vi "FileNamer_SM.vi"() -> ()   [LabVIEW 2024]
uses:
  TypeDefs/comic--cluster.ctl
  <userlib>/_OpenG.lib/array/array.llb/Remove Duplicates from 1D Array (String)__ogtk.vi
  <userlib>/_OpenG.lib/array/array.llb/Sort 1D Array (String)__ogtk.vi
  <userlib>/_OpenG.lib/file/file.llb/Strip Path Extension - String__ogtk.vi
  <userlib>/_OpenG.lib/array/array.llb/Remove Duplicates from 1D Array (DBL)__ogtk.vi
  <userlib>/_OpenG.lib/file/file.llb/Strip Path Extension - Path__ogtk.vi
  <userlib>/_OpenG.lib/array/array.llb/openg_array.lvlib
  <vilib>/httpClient/LabVIEWHTTPClient.lvlib
  <vilib>/addons/_JKI.lib/Serialization/JSON/JKI JSON Serialization.lvlib
  <userlib>/_OpenG.lib/file/file.llb/openg_file.lvlib
  <userlib>/_OpenG.lib/string/string.llb/openg_string.lvlib
panel:
  out "Available?":bool
  out "missing json":string
  out "missing current":string
  in  "Create New Folder":bool
  in  "json file path":path
  in  "Rename Available":bool
  out "json count":string
  out "current count":string
  in  "Rename Selected":bool
  in  "Delete from json":bool
  out "web cover":picture
  out "Local Cover":picture
  out "totals match":bool
  in  "Rename All":bool
  out "synced":bool
  in  "Rename Selected":bool
  in  "Folders":i32(listbox)
  in  "Parent Path":path
  in  "From json":i32(listbox)
  in  "Current":i32(listbox)
  in  "OK":bool
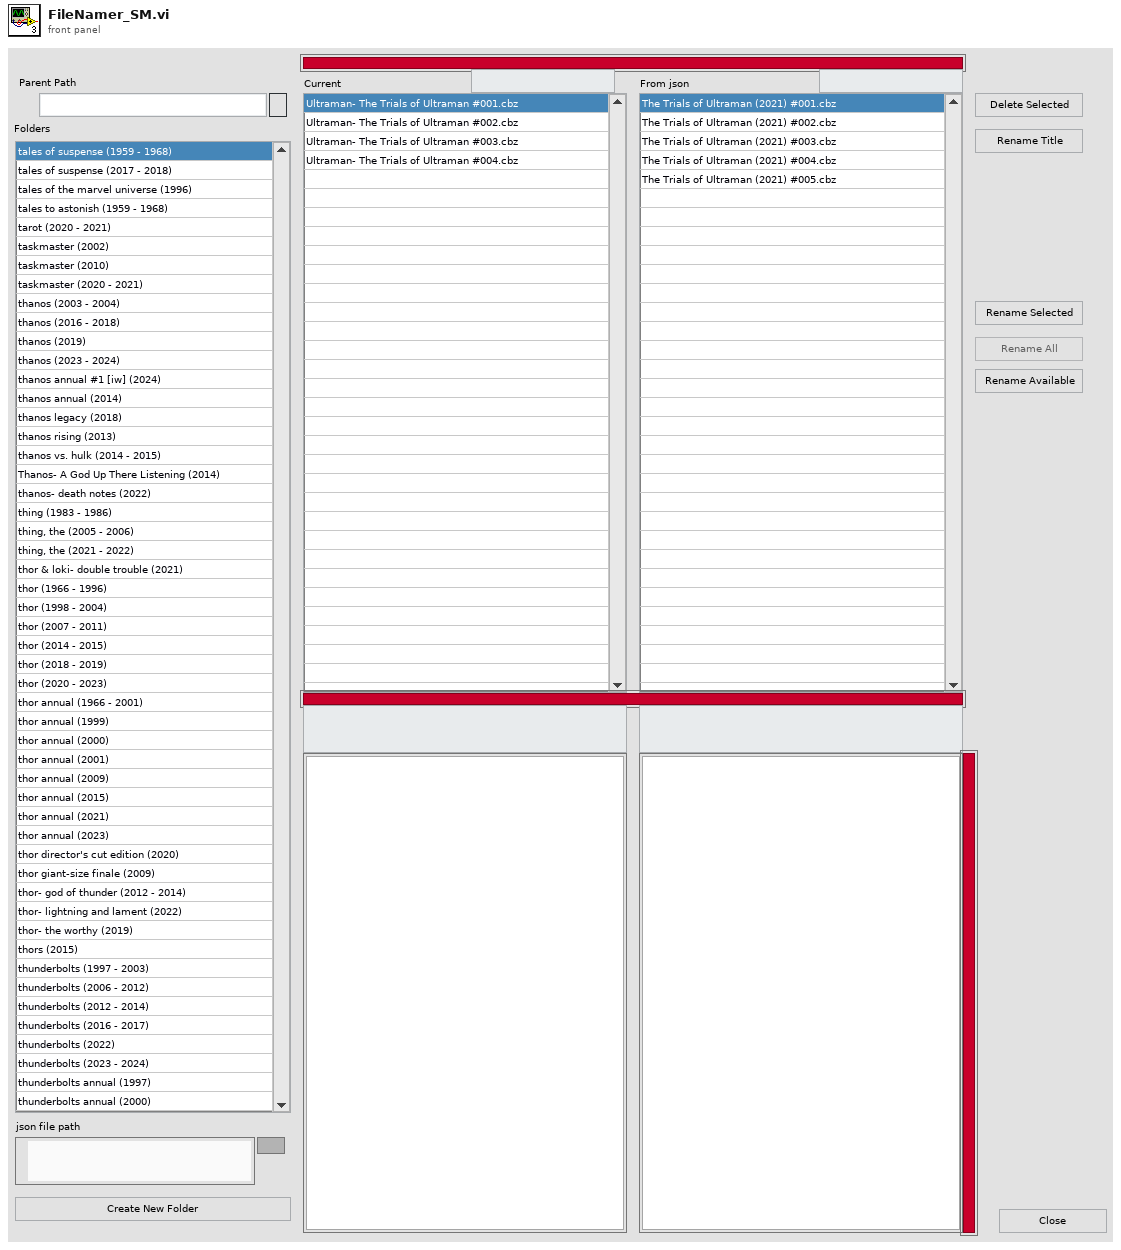
[diagram p1: front panel]
types:
  T1 = enum32{"Invalid", "Standard", "Closed", "Hidden", "Minimized", "Maximized"}
  T2 = enum32{"invalid app kind", "Development System", "Run Time System", "Student Edition", "Embedded LabVIEW", "Evaluation", "Custom"}
  T3 = enum16{"open", "replace", "create", "open or create", "replace or create", "replace or create with confirmation"}
  T4 = enum8{"Enabled", "Disabled", "Disabled and Grayed Out"}
  T5 = typedef "comic--cluster.ctl" = cluster{"id":i32, "digitalId":i32, "title":string, "issueNumber":i32, "variantDescription":string, "description":string, "modified":variant, "upc":string, "format":string, "pageCount":i32, "resourceURI":string, "urls":cluster{"type":string, "url":string}[], "series":cluster{"resourceURI":string, "name":string}, "dates":cluster{"type":string, "date":string}[], "prices":cluster{"price":dbl, "type":string}[], "thumbnail":cluster{"path":string, "extension":string}, "images":cluster{"path":string, "extension":string}[], "creators":cluster{"available":i32, "returned":i32, "collectionURI":string, "items":cluster{"resourceURI":string, "name":string, "role":string}[]}, "characters":cluster{"available":i32, "returned":i32, "collectionURI":string, "items":cluster{"resourceURI":string, "name":string}[]}, "stories":cluster{"available":i32, "returned":i32, "collectionURI":string, "items":cluster{"resourceURI":string, "name":string, "type":string}[]}, "events":cluster{"available":i32, "returned":i32, "collectionURI":string, "items":cluster{"resourceURI":string, "name":string}[]}}
  T6 = cluster{"Core":cluster{"Current VI Reference":refnum<vi>, "Close Panel on Exit?":bool}, "current folder":path, "comic jsons":T5[], "local working folder":path, "web working folder":path, "json present":bool, "display web":bool}
  T7 = cluster{"Current VI Reference":refnum<vi>, "Close Panel on Exit?":bool}
  T8 = typedef "comics.reply--cluster.ctl" = cluster{"code":i32, "status":string, "etag":string, "data":cluster{"offset":i32, "limit":i32, "total":i32, "count":i32, "results":T5[]}}
  T9 = typedef "imagedata.ctl" = cluster{"image type":i32, "image depth":i32, "image":u8[], "mask":u8[], "colors":u32[], "Rectangle":cluster{"left":i16, "top":i16, "right":i16, "bottom":i16}}
  T10 = typedef "LVBoundsTypeDef.ctl" = cluster{"Width":u32, "Height":u32}
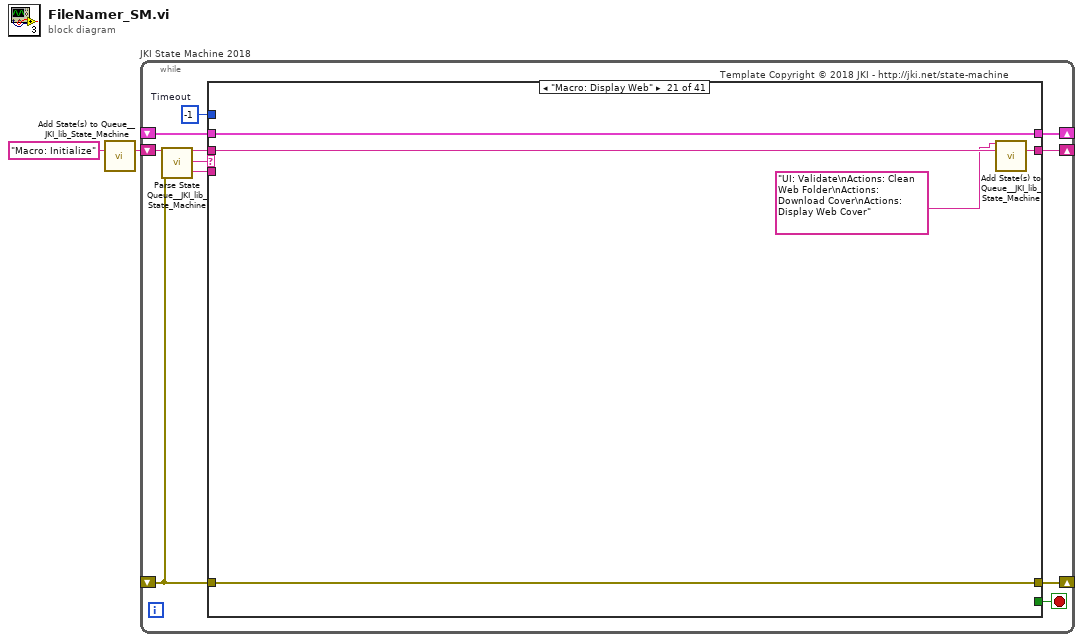
[diagram p0: block diagram]
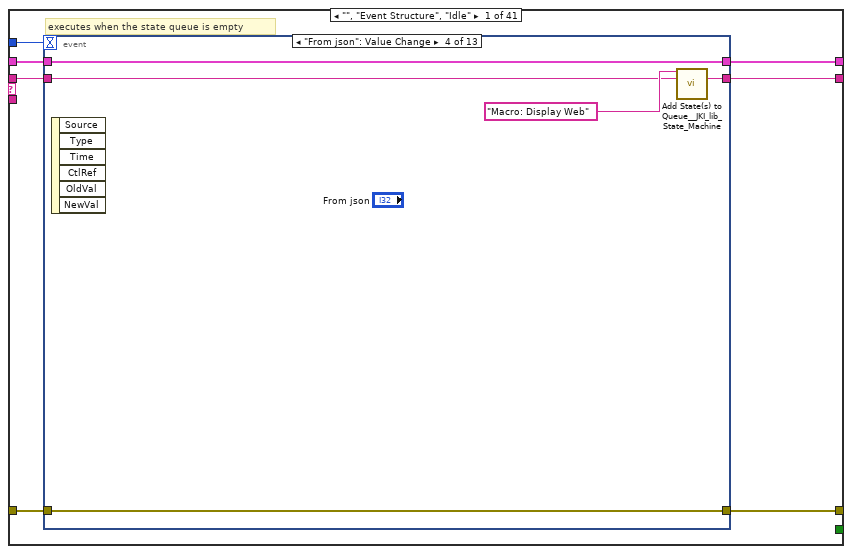
[diagram p2: hidden frame]
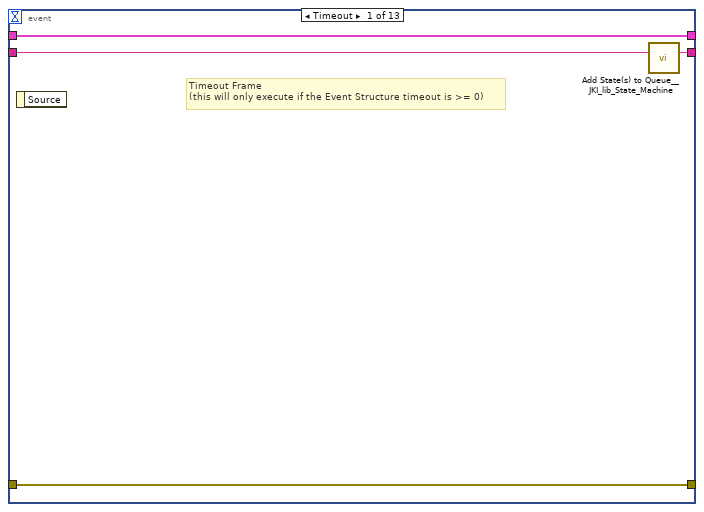
[diagram p3: hidden frame]
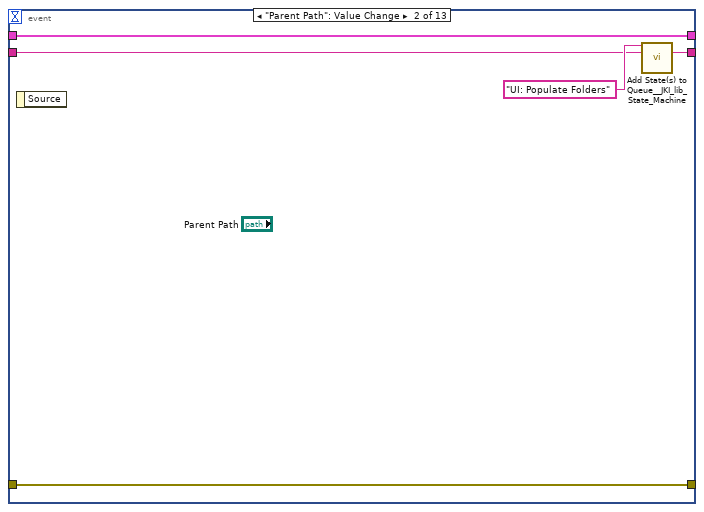
[diagram p4: hidden frame]
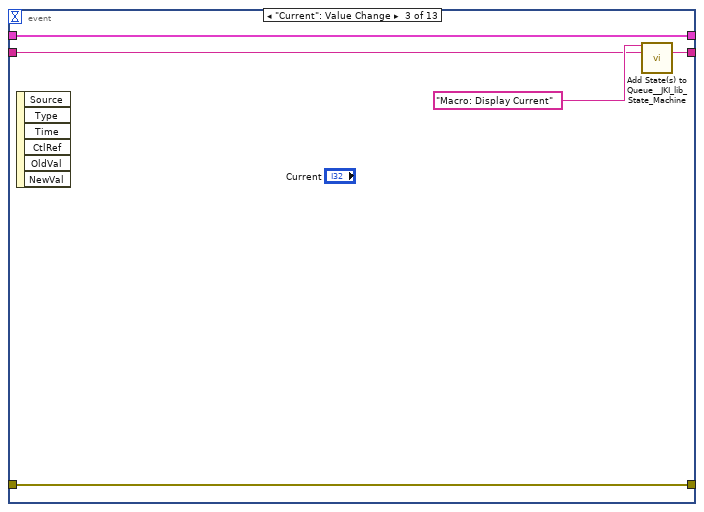
[diagram p5: hidden frame]
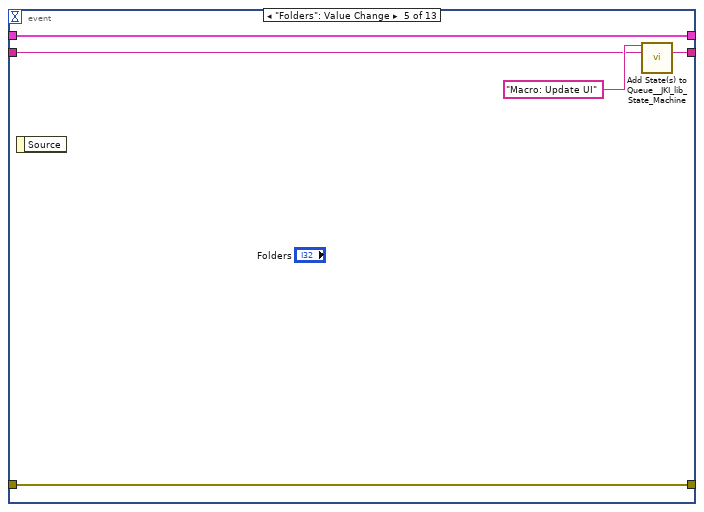
[diagram p6: hidden frame]
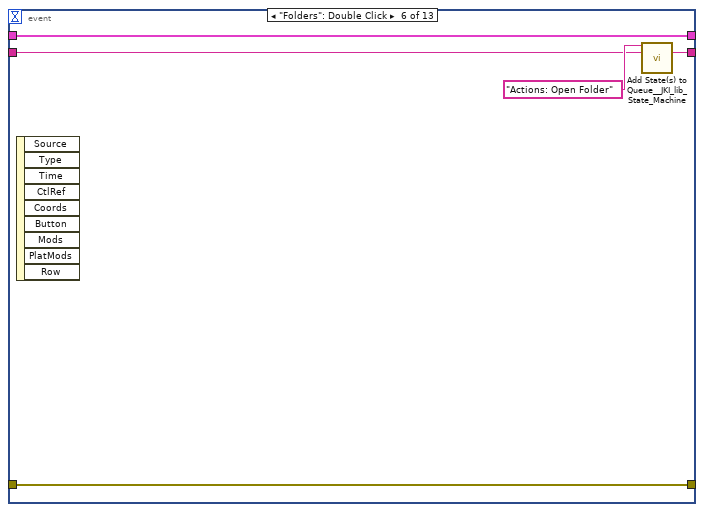
[diagram p7: hidden frame]
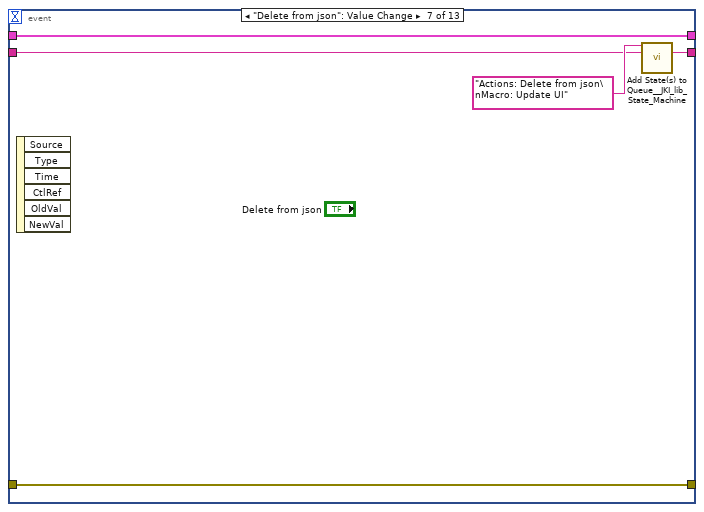
[diagram p8: hidden frame]
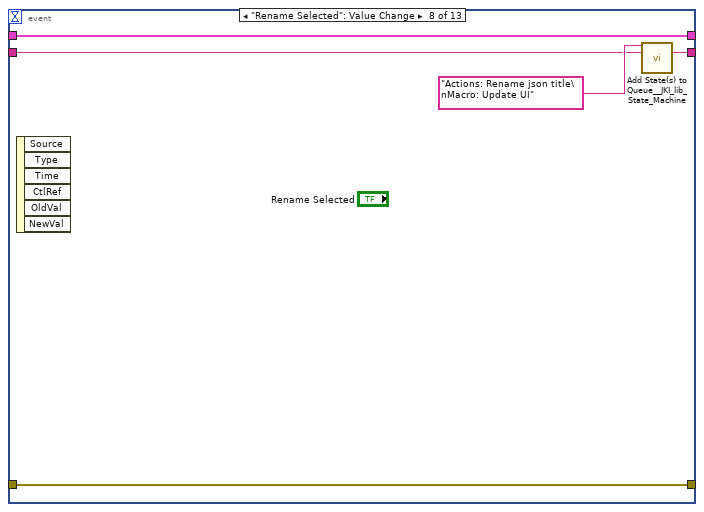
[diagram p9: hidden frame]
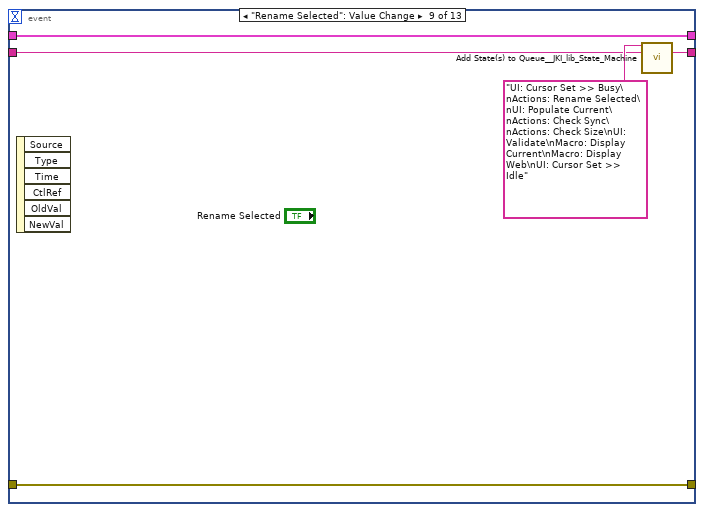
[diagram p10: hidden frame]
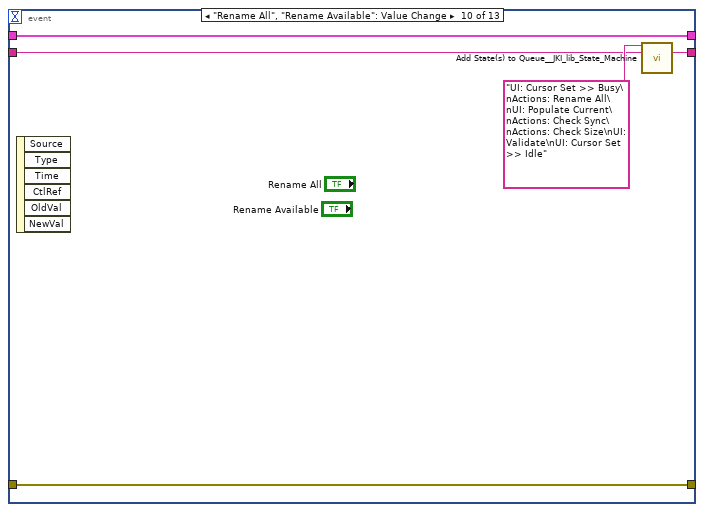
[diagram p11: hidden frame]
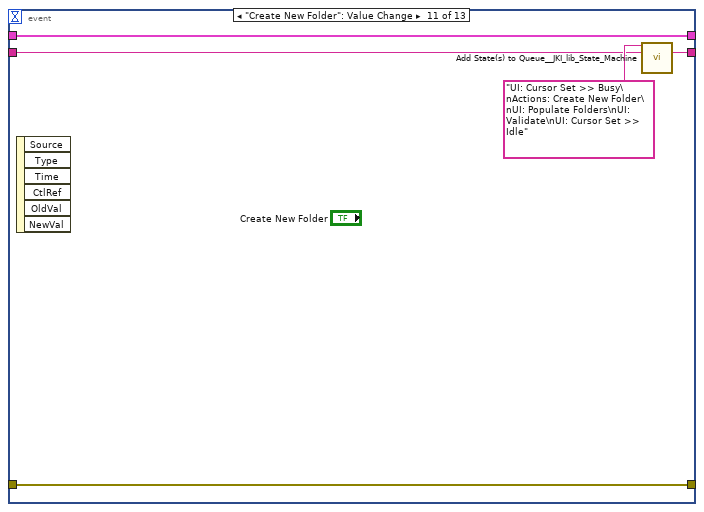
[diagram p12: hidden frame]
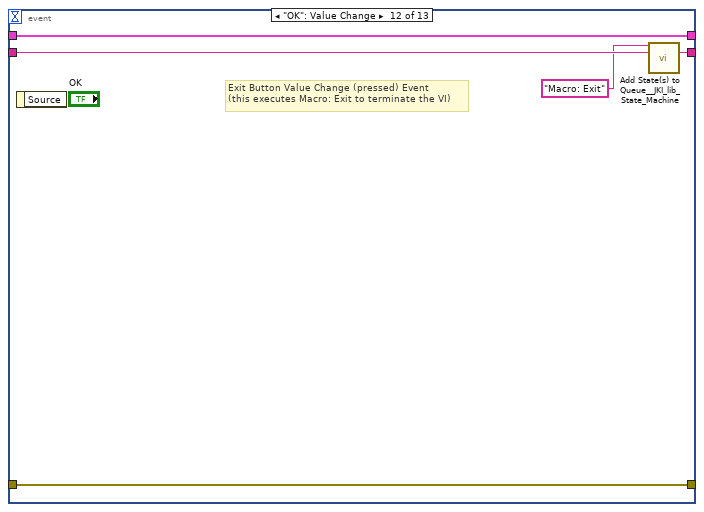
[diagram p13: hidden frame]
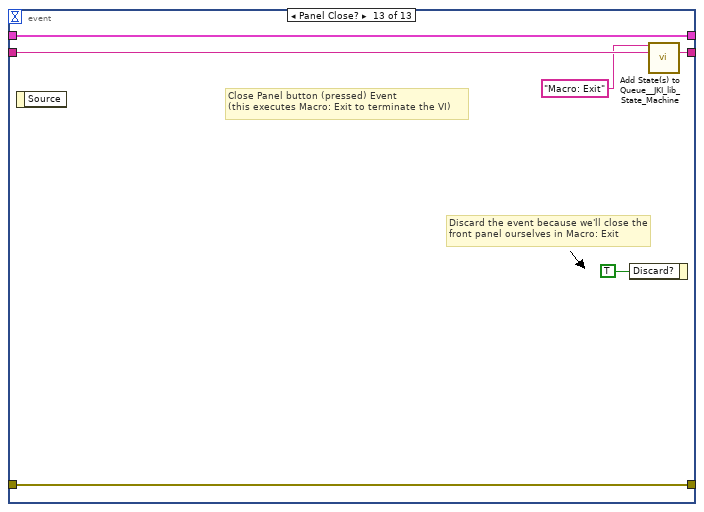
[diagram p14: hidden frame]
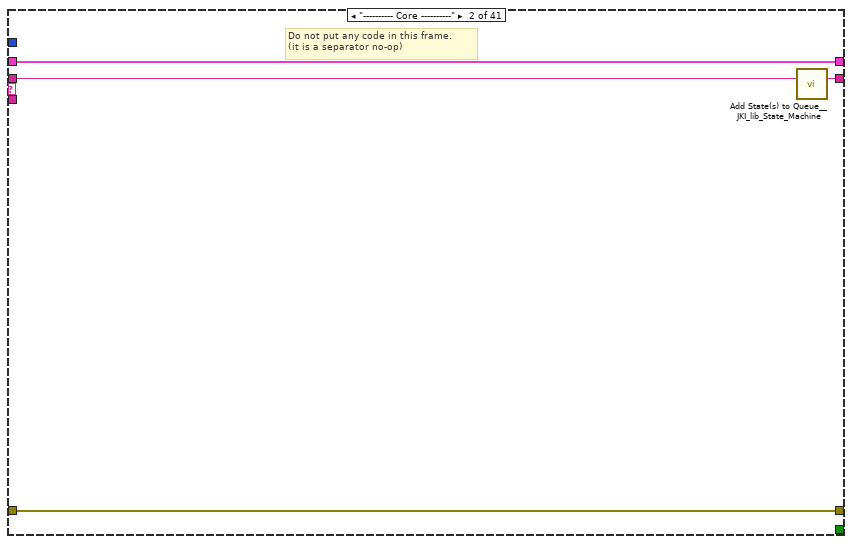
[diagram p15: hidden frame]
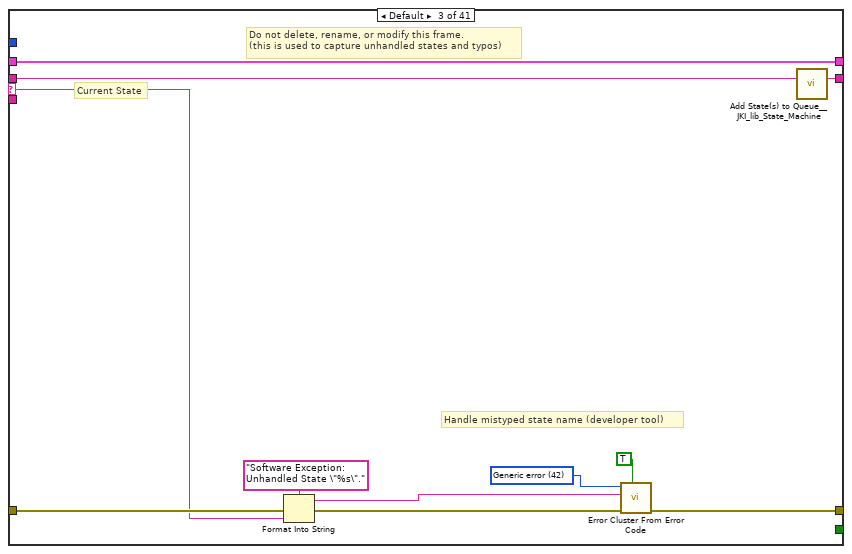
[diagram p16: hidden frame]
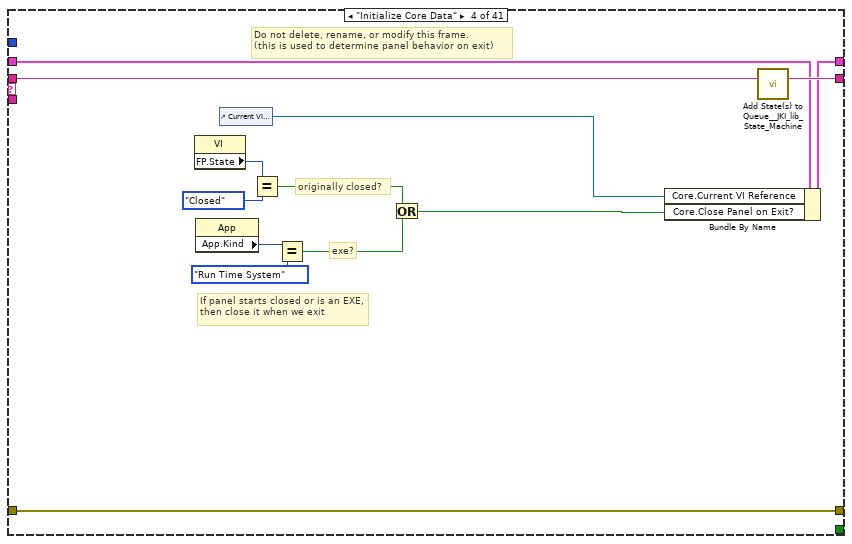
[diagram p17: hidden frame]
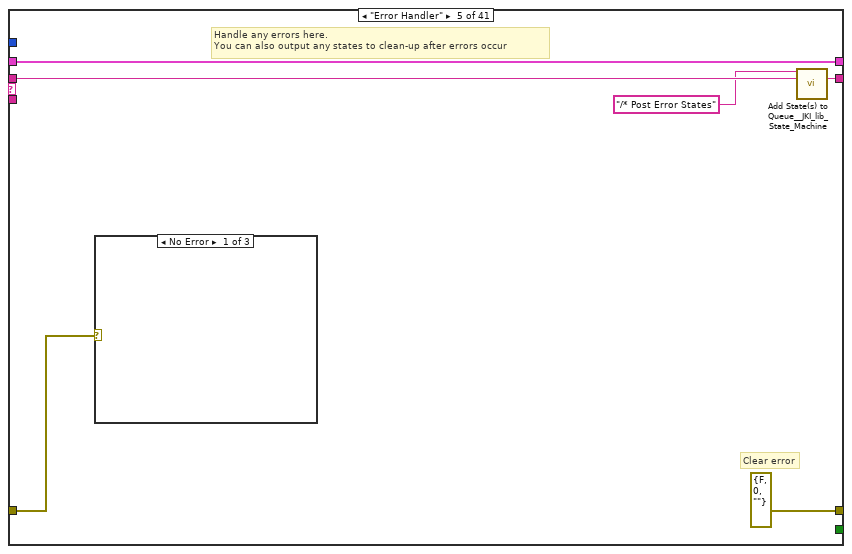
[diagram p18: hidden frame]
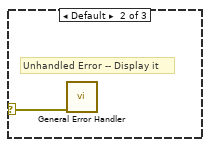
[diagram p19: hidden frame]
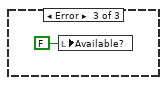
[diagram p20: hidden frame]
diagram:
  n1 = call <vilib>:"Add State(s) to Queue__JKI_lib_State_Machine.vi"("State(s) in (\"\")"="Macro: Initialize") -> ("States Out"=w2:string)  [unwired: 14 in]
  n2 = while "JKI State Machine 2018" {
    shift-right: [w6] -> _
    shift-left: _ -> [w5]
    shift-right: [w9] -> _
    shift-left: _ -> [w3]
    shift-right: [w8] -> _
    shift-left: w2 -> [w10]
    stop <- w7 stop-if-true
    w4 = -1  # Timeout
    # "Template Copyright © 2018 JKI - http://jki.net/state-machine"
    n3 = call <vilib>:"Parse State Queue__JKI_lib_State_Machine.vi"("State Queue"=w10, "Error In (no error)"=w3) -> ("Remaining States"=w12:string, "Current State"=w13:string, "Arguments"=w11:string)  [unwired: 11 in]
    n4 = case shown="\"Macro: Display Web\"" w13 {
      selector: w13 -> [_ _ w90 _ _ _ _ _ _ _ _ _ _ _ _ _ _ _ _ _ _ _ _ _ _ _ _ _ _ _ _ _ _ _ _ _ _ _ _ _ _]
      tunnel: w12 -> [w20 w89 w94 w113 w119 w126 w130 w141 w147 w151 w162 w171 w201 w237 w246 w267 w285 w296 w365 w370 w375 w380 w385 w395 w399 w405 w426 w487 w518 w527 w567 w612 w645 w672 w678 w684 w702 w721 w744 w758 w780]
      tunnel: w11 -> [_ _ _ _ _ _ _ _ _ _ _ _ _ _ _ _ w280 w290 _ _ _ _ _ _ _ _ _ _ _ _ _ _ _ _ _ _ _ _ _ _ _]
      tunnel: w5 -> [w18 w86 w92 w106 w116 w124 w127 _ w142 w148 w156 w165 w196 w231 w244 w262 w283 w292 w362 w367 w372 w377 w382 w392 w396 w403 w423 w485 w513 w525 w558 w610 w643 w662 w674 w680 w693 w715 w738 w755 w777]
      tunnel: [w17 w87 w96 w110 errorcluster {"status"=FALSE, "code"=0, "source"=""} ("error out") w123 w128 w138 w143 w149 w157 w166 w199 w224 w239 w247 w281 w293 w363 w368 w373 w378 w383 w393 w397 w400 w424 w484 w496 w523 w559 w592 w631 w663 w676 w682 w694 w716 w739 w753 w775] -> w9
      tunnel: w3 -> [w16 w87 w95 w110 w114 w123 w128 w138 w144 w149 w160 w168 w198 w226 w242 w250 w282 w294 w363 w368 w373 w378 w383 w393 w397 w401 w424 w478 w509 w522 w562 w608 w629 w658 w675 w681 w695 w719 w737 w756 w778]
      tunnel: [w19 w88 w93 w112 w118 w125 w129 w140 w146 w150 w161 w170 w200 w236 w245 w266 w284 w295 w364 w369 w374 w379 w384 w394 w398 w404 w425 w486 w517 w526 w566 w611 w644 w671 w677 w683 w701 w720 w743 w757 w779] -> w8
      tunnel: [_ _ _ _ _ TRUE _ _ _ _ _ _ _ _ _ _ _ _ _ _ _ _ _ _ _ _ _ _ _ _ _ _ _ _ _ _ _ _ _ _ _] -> w7
      tunnel: [w15 w86 w92 w111 w116 w124 w127 w139 w142 w148 w156 w165 w195 w230 w244 w261 w283 w292 w362 w367 w372 w377 w382 w392 w396 w403 w423 w485 w512 w524 w557 w610 w643 w662 w674 w680 w692 w715 w738 w755 w777] -> w6
      tunnel: w4 -> [w14 _ _ _ _ _ _ _ _ _ _ _ _ _ _ _ _ _ _ _ _ _ _ _ _ _ _ _ _ _ _ _ _ _ _ _ _ _ _ _ _]
      frame "", "Event Structure", "Idle" {
        # "executes when the state queue is empty"
        n5 = event shown="[3] \"From json\": Value Change" {
          selector: _ -> [_ _ _ _ _ _ _ _ _ _ _ _ _]
          dyn-events: _ -> [_ _ _ _ _ _ _ _ _ _ _ _ _]
          timeout: w14 -> [_ _ _ _ _ _ _ _ _ _ _ _ _]
          tunnel: w20 -> [w24 w27 w32 w37 w42 w47 w52 w57 w62 w67 w72 w79 w85]
          tunnel: [w23 w26 w31 w36 w41 w46 w51 w56 w61 w66 w71 w78 w84] -> w19
          tunnel: w18 -> [w21 w28 w33 w38 w43 w48 w53 w58 w63 w68 w73 w76 w82]
          tunnel: [w22 w25 w30 w35 w40 w45 w50 w55 w60 w65 w70 w77 w83] -> w17
          tunnel: w16 -> [w22 w25 w30 w35 w40 w45 w50 w55 w60 w65 w70 w77 w83]
          tunnel: [w21 w28 w33 w38 w43 w48 w53 w58 w63 w68 w73 w76 w82] -> w15
          event Timeout {
            # "Timeout Frame\n(this will only execute if the Event Structure timeout is >= 0)"
            n6 = event-data() -> ()  [unwired: 1 in, 1 out]
            n7 = call <vilib>:"Add State(s) to Queue__JKI_lib_State_Machine.vi"("State(s) in (\"\")"=w24) -> ("States Out"=w23:string)  [unwired: 14 in]
          }
          event "Parent Path": Value Change {
            n8 = event-data() -> ()  [unwired: 1 in, 1 out]
            n9 = call <vilib>:"Add State(s) to Queue__JKI_lib_State_Machine.vi"("State(s) in Front (\"\")"="UI: Populate Folders", "State(s) in (\"\")"=w27) -> ("States Out"=w26:string)  [unwired: 13 in]
          }
          event "Current": Value Change {
            n10 = event-data() -> ()  [unwired: 1 in, 6 out]
            n11 = call <vilib>:"Add State(s) to Queue__JKI_lib_State_Machine.vi"("State(s) in Front (\"\")"="Macro: Display Current", "State(s) in (\"\")"=w32) -> ("States Out"=w31:string)  [unwired: 13 in]
          }
          event "From json": Value Change {
            n12 = event-data() -> ()  [unwired: 1 in, 6 out]
            n13 = call <vilib>:"Add State(s) to Queue__JKI_lib_State_Machine.vi"("State(s) in Front (\"\")"="Macro: Display Web", "State(s) in (\"\")"=w37) -> ("States Out"=w36:string)  [unwired: 13 in]
          }
          event "Folders": Value Change {
            n14 = event-data() -> ()  [unwired: 1 in, 1 out]
            n15 = call <vilib>:"Add State(s) to Queue__JKI_lib_State_Machine.vi"("State(s) in Front (\"\")"="Macro: Update UI", "State(s) in (\"\")"=w42) -> ("States Out"=w41:string)  [unwired: 13 in]
          }
          event "Folders": Double Click {
            n16 = event-data() -> ()  [unwired: 1 in, 9 out]
            n17 = call <vilib>:"Add State(s) to Queue__JKI_lib_State_Machine.vi"("State(s) in Front (\"\")"="Actions: Open Folder", "State(s) in (\"\")"=w47) -> ("States Out"=w46:string)  [unwired: 13 in]
          }
          event "Delete from json": Value Change {
            n18 = event-data() -> ()  [unwired: 1 in, 6 out]
            n19 = call <vilib>:"Add State(s) to Queue__JKI_lib_State_Machine.vi"("State(s) in Front (\"\")"="Actions: Delete from json\nMacro: Update UI", "State(s) in (\"\")"=w52) -> ("States Out"=w51:string)  [unwired: 13 in]
          }
          event "Rename Selected": Value Change {
            n20 = event-data() -> ()  [unwired: 1 in, 6 out]
            n21 = call <vilib>:"Add State(s) to Queue__JKI_lib_State_Machine.vi"("State(s) in Front (\"\")"="Actions: Rename json title\nMacro: Update UI", "State(s) in (\"\")"=w57) -> ("States Out"=w56:string)  [unwired: 13 in]
          }
          event "Rename Selected": Value Change {
            n22 = event-data() -> ()  [unwired: 1 in, 6 out]
            n23 = call <vilib>:"Add State(s) to Queue__JKI_lib_State_Machine.vi"("State(s) in Front (\"\")"="UI: Cursor Set >> Busy\nActions: Rename Selected\nUI: Populate Current\nActions: Check Sync\nActions: Check Size\nUI: Validate\nMacro: Display Current\nMacro: Display Web\nUI: Cursor Set >> Idle", "State(s) in (\"\")"=w62) -> ("States Out"=w61:string)  [unwired: 13 in]
          }
          event "Rename All", "Rename Available": Value Change {
            n24 = event-data() -> ()  [unwired: 1 in, 6 out]
            n25 = call <vilib>:"Add State(s) to Queue__JKI_lib_State_Machine.vi"("State(s) in Front (\"\")"="UI: Cursor Set >> Busy\nActions: Rename All\nUI: Populate Current\nActions: Check Sync\nActions: Check Size\nUI: Validate\nUI: Cursor Set >> Idle", "State(s) in (\"\")"=w67) -> ("States Out"=w66:string)  [unwired: 13 in]
          }
          event "Create New Folder": Value Change {
            n26 = event-data() -> ()  [unwired: 1 in, 6 out]
            n27 = call <vilib>:"Add State(s) to Queue__JKI_lib_State_Machine.vi"("State(s) in Front (\"\")"="UI: Cursor Set >> Busy\nActions: Create New Folder\nUI: Populate Folders\nUI: Validate\nUI: Cursor Set >> Idle", "State(s) in (\"\")"=w72) -> ("States Out"=w71:string)  [unwired: 13 in]
          }
          event "OK": Value Change {
            # "Exit Button Value Change (pressed) Event\n(this executes Macro: Exit to terminate the VI)"
            n28 = event-data() -> ()  [unwired: 1 in, 1 out]
            n29 = call <vilib>:"Add State(s) to Queue__JKI_lib_State_Machine.vi"("State(s) in Front (\"\")"="Macro: Exit", "State(s) in (\"\")"=w79) -> ("States Out"=w78:string)  [unwired: 13 in]
          }
          event Panel Close? {
            # "Discard the event because we'll close the front panel ourselves in Macro: Exit"
            # "Close Panel button (pressed) Event\n(this executes Macro: Exit to terminate the VI)"
            n30 = event-data() -> ()  [unwired: 1 in, 1 out]
            n31 = event-data("Discard?"=TRUE) -> ()  [unwired: 1 in, 1 out]
            n32 = call <vilib>:"Add State(s) to Queue__JKI_lib_State_Machine.vi"("State(s) in Front (\"\")"="Macro: Exit", "State(s) in (\"\")"=w85) -> ("States Out"=w84:string)  [unwired: 13 in]
          }
        }
      }
      frame "---------- Core ----------" {
        # "Do not put any code in this frame.\n(it is a separator no-op)"
        n33 = call <vilib>:"Add State(s) to Queue__JKI_lib_State_Machine.vi"("State(s) in (\"\")"=w89) -> ("States Out"=w88:string)  [unwired: 14 in]
      }
      frame Default {
        w99 = 42 items=["No error", "Argument error", "Memory is full", "Out of zone", "End of file", "File already open", "Generic file I/O error", "File not found", "File permission error", "Disk is full", "Duplicate path", "Too many files open", "System feature not enabled", "Resource file not found", "Cannot add resource", "Resource not found", "Image not found", "Image memory error", "Pen does not exist", "Config type invalid", "Config token not found", "Config parse error", "Config memory error", "Bad external code format", "Bad external code offset", "External code not present", "Null window", "Destroy window error", "Null menu", "Print aborted", "Bad print record", "Print driver error", "Windows error during printing", "Memory error during printing", "Print dialog error", "Generic print error", "Invalid device refnum", "Device not found", "Device parameter error", "Device unit error", "Cannot open device", "Device call aborted", "Generic error", "Cancelled by user", "Object ID too low", "Object ID too high", "Object not in heap", "Unknown heap", "Unknown object (invalid DefProc)", "Unknown object (DefProc not in table)", "Message out of range", "Invalid (null) method", "Unknown message", "Manager call not supported", "Bad address", "Network operation in progress", "Network operation timed out", "Connection is busy", "Network attribute not supported", "Network error", "Address in use", "System out of memory", "Connection aborted", "Connection refused", "Not connected", "Already connected", "Connection closed", "Initialization error (interapplication manager)", "Bad occurrence", "Wait on unbound occurrence handler", "Occurrence queue overflow", "Datalog type conflict", "Unused", "Unrecognized type (interapplication manager)", "Memory corrupt", "Failed to make temporary DLL", "Old CIN version", "Drag socket not found", "Failed to load drop-object", "Failed to register OLE object", "Failed to release OLE object", "Format specifier type mismatch", "Unknown format specifier", "Too few format specifiers", "Too many format specifiers", "Scan failed", "Newer CIN version", "Error converting to variant", "Runtime menu error", "Password tampered", "Variant attribute not found", "Incompatible variant data type", "Event data is not available", "Event Store is not present", "Occurrence is not found", "Event Queue is not created", "Event info is not available", "Refnum passed is NULL", "Error retrieving Class GUID", "Error retrieving CoClass GUID", "Error retrieving TypeLib GUID.", "Bad built application magic bytes.", "Specific driver is different from the specific driver associated with the Logical Name.", "There is no session opened to the class driver.", "Max Error", "MAX - Error with config objects", "MAX - Error loading configuration", "MAX - Group not supported"]
        # "Current State"
        # "Do not delete, rename, or modify this frame.\n(this is used to capture unhandled states and typos)"
        # "Handle mistyped state name (developer tool)"
        n34 = Format Into String(format string="Software Exception: Unhandled State \"%s\"." ("message"), error in=w95, w90) -> (resulting string=w98:string, error out=w97:errorcluster)  [unwired: 1 in]
        n35 = call <vilib>:"Error Cluster From Error Code.vi"("show call chain? (False)"=TRUE, "error in (no error)"=w97, "error message (\"\")"=w98, "error code (0)"=w99) -> ("error out"=w96:errorcluster)  [unwired: 5 in]
        n36 = call <vilib>:"Add State(s) to Queue__JKI_lib_State_Machine.vi"("State(s) in (\"\")"=w94) -> ("States Out"=w93:string)  [unwired: 14 in]
      }
      frame "Initialize Core Data" {
        # "Do not delete, rename, or modify this frame.\n(this is used to determine panel behavior on exit)"
        # "originally closed?"
        # "exe?"
        # "If panel starts closed or is an EXE, then close it when we exit"
        n37 = property class="VI"() -> ("FP.State"=w103:T1)  [unwired: 2 in, 2 out]
        n38 = property class="App"() -> ("App.Kind"=w109:T2)  [unwired: 2 in, 2 out]
        n39 = control-ref of="Current VI Reference"() -> (w104:refnum<vi>)
        n40 = Equal?(x=w103, y=T1."Closed" ("Front Panel Window:State")) -> (x = y?=w101:bool)
        n41 = Equal?(x=w109, y=T2."Run Time System" ("Application:Kind")) -> (x = y?=w107:bool)
        n42 = Or(x=w101, y=w107) -> (x .or. y?=w105:bool)
        n43 = Bundle By Name(cluster=w106, "Core.Current VI Reference"=w104, "Core.Close Panel on Exit?"=w105) -> (w111:T6)
        n44 = call <vilib>:"Add State(s) to Queue__JKI_lib_State_Machine.vi"("State(s) in (\"\")"=w113) -> ("States Out"=w112:string)  [unwired: 14 in]
      }
      frame "Error Handler" {
        # "Handle any errors here.\nYou can also output any states to clean-up after errors occur"
        # "Clear error"
        n45 = case shown="No Error" w114 {
          selector: w114 -> [_ w120 _]
          frame No Error {
          }
          frame Default {
            # "Unhandled Error -- Display it"
            n46 = call <vilib>:"General Error Handler.vi"("error in (no error)"=w120) -> ()  [unwired: 10 in, 5 out]
          }
          frame Error {
            n47 = local write "Available?"(FALSE ("Available?")) -> ()
          }
        }
        n48 = call <vilib>:"Add State(s) to Queue__JKI_lib_State_Machine.vi"("State(s) in Front (\"\")"="/* Post Error States", "State(s) in (\"\")"=w119) -> ("States Out"=w118:string)  [unwired: 13 in]
      }
      frame "Exit" {
        # "Do not put any code in this frame.\n(No errors that occur here will be handled.)"
        n49 = call <vilib>:"Add State(s) to Queue__JKI_lib_State_Machine.vi"("State(s) in (\"\")"=w126) -> ("States Out"=w125:string)  [unwired: 14 in]
      }
      frame "---------- Data ----------" {
        # "Do not put any code in this frame.\n(It is a separator no-op. You can make a copy of this frame to create a new Data frame)"
        n50 = call <vilib>:"Add State(s) to Queue__JKI_lib_State_Machine.vi"("State(s) in (\"\")"=w130) -> ("States Out"=w129:string)  [unwired: 14 in]
      }
      frame "Data: Initialize" {
        w131 = TRUE  # display web
        w132 = FALSE  # json present
        w133 = path "FileName_web"  # web working folder
        w134 = path "FileName_local"  # local working folder
        w135 = T5[] []  # comic jsons
        w136 = T7 {"Current VI Reference"=refnum, "Close Panel on Exit?"=FALSE}  # Core
        w137 = path ""  # current folder
        # "Data names and types of shift register data are defined by this bundle."
        # "Initialize the shift-register data, here.\n(data names are defined by what you wire into the bundle function)"
        n51 = Bundle("Core"=w136, "current folder"=w137, "comic jsons"=w135, "local working folder"=w134, "web working folder"=w133, "json present"=w132, "display web"=w131) -> (w139:T6)  [unwired: 1 in]
        n52 = call <vilib>:"Add State(s) to Queue__JKI_lib_State_Machine.vi"("State(s) in (\"\")"=w141) -> ("States Out"=w140:string)  [unwired: 14 in]
      }
      frame "Data: Cleanup" {
        # "Cleanup any data and references, here.\n(this is called automatically, by the Macro: Exit)"
        n53 = Unbundle By Name(w142) -> ("Core.Current VI Reference"=w145:refnum<vi>)
        n54 = Close Reference(reference=w145, error in (no error)=w144) -> (error out=w143:errorcluster)
        n55 = call <vilib>:"Add State(s) to Queue__JKI_lib_State_Machine.vi"("State(s) in (\"\")"=w147) -> ("States Out"=w146:string)  [unwired: 14 in]
      }
      frame "---------- UI ----------" {
        # "Do not put any code in this frame.\n(It is a separator no-op. You can make a copy of this frame to create a new UI frame)"
        n56 = call <vilib>:"Add State(s) to Queue__JKI_lib_State_Machine.vi"("State(s) in (\"\")"=w151) -> ("States Out"=w150:string)  [unwired: 14 in]
      }
      frame "UI: Reset Selections" {
        w155 = 0 ("Value (Signaling)")
        n57 = Unbundle By Name(w156) -> ("json present"=w154:bool)
        n58 = Select(t=w155, s=w154, f=-1) -> (s? t:f=w152:i32)
        n59 = property on="Current" class="LstBox (strict)"(error in=w160, "Val(Sgnl)"=w155) -> (error out=w158:errorcluster)  [unwired: 1 in, 1 out]
        n60 = property on="From json" class="LstBox (strict)"(error in=w160, "Val(Sgnl)"=w152) -> (error out=w159:errorcluster)  [unwired: 1 in, 1 out]
        n61 = Merge Errors(w158, w159) -> (w157:errorcluster)
        n62 = call <vilib>:"Add State(s) to Queue__JKI_lib_State_Machine.vi"("State(s) in (\"\")"=w162) -> ("States Out"=w161:string)  [unwired: 14 in]
      }
      frame "UI: Validate" {
        n63 = Unbundle By Name(w165) -> ("json present"=w164:bool)
        n64 = case shown="True" w164 {
          tunnel: [w172 w189] -> w169
          tunnel: [w172 w178] -> w163
          frame False {
            w172 = T4."Disabled and Grayed Out" ("Disabled")
          }
          frame True {
            w180 = T4."Disabled and Grayed Out" ("Disabled")
            w179 = T4."Enabled" ("Disabled")
            n65 = local read "totals match"() -> (w188:bool)
            n66 = local read "From json"() -> (w183:i32)
            n67 = local read "synced"() -> (w187:bool)
            n68 = property on="Current" class="LstBox (strict)"() -> ("Item Names"=w184:string[])  [unwired: 2 in, 2 out]
            n69 = local read "Current"() -> (w185:i32)
            n70 = property on="From json" class="LstBox (strict)"() -> ("Item Names"=w177:string[])  [unwired: 2 in, 2 out]
            n71 = Compound Arithmetic op=AND(w188, invert w187) -> (w186:bool)
            n72 = Index Array(array=w184, index=w185) -> (element=w182:string)
            n73 = Index Array(array=w177, index=w183) -> (element=w181:string)
            n74 = call-poly <userlib>:"Remove Duplicates from 1D Array__ogtk.vi"("Input Array"=w177) -> ("indices of removed elements"=w176:i32[])  [unwired: 1 out]
            n75 = Empty Array?(array=w176) -> (empty?=w174:bool)
            n76 = Equal?(x=w182, y=w181) -> (x = y?=w175:bool)
            n77 = And(x=w175, y=w174) -> (x .and. y?=w173:bool)
            n78 = Select(t=w179, s=w186, f=w180) -> (s? t:f=w189:T4)
            n79 = Select(t=w180, s=w173, f=w179) -> (s? t:f=w178:T4)
          }
        }
        n80 = property on="Rename All" class="Bool"(error in=w168, "DisabledEnum"=w169) -> (error out=w167:errorcluster)  [unwired: 1 in, 1 out]
        n81 = property on="Rename Selected" class="Bool"(error in=w167, "DisabledEnum"=w163) -> (error out=w166:errorcluster)  [unwired: 1 in, 1 out]
        n82 = property on="Rename Available" class="Bool"("DisabledEnum"=w163) -> ()  [unwired: 2 in, 2 out]
        n83 = call <vilib>:"Add State(s) to Queue__JKI_lib_State_Machine.vi"("State(s) in (\"\")"=w171) -> ("States Out"=w170:string)  [unwired: 14 in]
      }
      frame "UI: Populate From json" {
        n84 = Unbundle By Name(w196) -> ("comic jsons"=w197:T5[], "json present"=w194:bool)
        n85 = case shown="True" w194 {
          tunnel: [_ w208] -> w191
          tunnel: w197 -> [_ w206]
          tunnel: w196 -> [w202 w205]
          tunnel: [w202 w203] -> w195
          frame False {
          }
          frame True {
            n86 = for {
              tunnel: w206 -> [w218] mode=indexing
              tunnel: [w213] -> w209 mode=indexing
              n87 = Unbundle By Name(w218) -> ("title"=w217:string)
              n88 = call "BufferComicNameNumber.vi"("string in"=w217) -> ("buffered number string"=w216:string)  [unwired: 10 in]
              n89 = Concatenate Strings(w216, ".cbz" ("string")) -> (w214:string)
              n90 = call "remove.invalid.chars.vi"("string in"=w214) -> ("string out"=w213:string)
            }
            n91 = call-poly <userlib>:"Sort Array__ogtk.vi"("Array in"=w209) -> ("Sorted Pointers"=w207:i32[], "Sorted Array out"=w208:string[])  [unwired: 9 in]
            n92 = for {
              tunnel: w207 -> [w211] mode=indexing
              tunnel: w206 -> [w212]
              tunnel: [w210] -> w204 mode=indexing
              n93 = Index Array(array=w212, index=w211) -> (element=w210:T5)
            }
            n94 = Bundle By Name(cluster=w205, "comic jsons"=w204) -> (w203:T6)
          }
        }
        n95 = Array Size(array=w191) -> (size(s)=w192:i32)
        n96 = Format Into String(format string="Total Count: %d", w192) -> (resulting string=→"json count":string)  [unwired: 2 in, 1 out]
        n97 = property on="From json" class="LstBox (strict)"(error in=w198, "Item Names"=w191) -> (error out=w199:errorcluster)  [unwired: 1 in, 1 out]
        n98 = call <vilib>:"Add State(s) to Queue__JKI_lib_State_Machine.vi"("State(s) in (\"\")"=w201) -> ("States Out"=w200:string)  [unwired: 14 in]
      }
      frame "UI: Populate Current" {
        n99 = local read "Parent Path"() -> (w233:path)
        n100 = property on="Folders" class="LstBox (strict)"(error in=w226) -> (error out=w227:errorcluster, "Item Names"=w235:string[])  [unwired: 1 in, 1 out]
        n101 = local read "Folders"() -> (w234:i32)
        n102 = Index Array(array=w235, index=w234) -> (element=w232:string)
        n103 = Build Path(base path=w233, name or relative path=w232) -> (appended path=w229:path)
        n104 = Bundle By Name(cluster=w231, "current folder"=w229) -> (w230:T6)
        n105 = List Folder(path=w229, pattern="*.cbz", error in=w227) -> (filenames=w223:string[], error out=w225:errorcluster)  [unwired: 1 in, 2 out]
        n106 = Sort 1D Array(array=w223) -> (sorted array=w222:string[])
        n107 = Array Size(array=w222) -> (size(s)=w220:i32)
        n108 = property on="Current" class="LstBox (strict)"(error in=w225, "Item Names"=w222) -> (error out=w224:errorcluster)  [unwired: 1 in, 1 out]
        n109 = Format Into String(format string="Total Count: %d", w220) -> (resulting string=→"current count":string)  [unwired: 2 in, 1 out]
        n110 = call <vilib>:"Add State(s) to Queue__JKI_lib_State_Machine.vi"("State(s) in (\"\")"=w237) -> ("States Out"=w236:string)  [unwired: 14 in]
      }
      frame "UI: Populate Folders" {
        n111 = local read "Parent Path"() -> (w243:path)
        n112 = List Folder(path=w243, error in=w242) -> (folder names=w241:string[], error out=w240:errorcluster)  [unwired: 2 in, 2 out]
        n113 = property on="Folders" class="LstBox (strict)"(error in=w240, "Item Names"=w241, "Val(Sgnl)"=0 ("Value (Signaling)")) -> (error out=w239:errorcluster)  [unwired: 1 in, 1 out]
        n114 = call <vilib>:"Add State(s) to Queue__JKI_lib_State_Machine.vi"("State(s) in (\"\")"=w246) -> ("States Out"=w245:string)  [unwired: 14 in]
      }
      frame "UI: Initialize" {
        w264 = path "FileName_web"  # web working folder
        w265 = path "FileName_local"  # local working folder
        # "Initialize the User Interface, here.\n(this is called automatically, by the Macro: Init)"
        n115 = Temporary Directory() -> (w263:path)
        n116 = Build Path(base path=w263, name or relative path=w265) -> (appended path=w252:path)
        n117 = Build Path(base path=w263, name or relative path=w264) -> (appended path=w260:path)
        n118 = call <vilib>:"Check if File or Folder Exists.vi"("error in (no error)"=w250, "path"=w252) -> ("error out"=w255:errorcluster, "file or folder exists?"=w253:bool, "dup path"=w254:path)  [unwired: 7 in]
        n119 = call <vilib>:"Check if File or Folder Exists.vi"("error in (no error)"=w250, "path"=w260) -> ("error out"=w257:errorcluster, "file or folder exists?"=w259:bool, "dup path"=w258:path)  [unwired: 7 in]
        n120 = case shown="True" w253 {
          tunnel: w254 -> [w271 w273]
          tunnel: w255 -> [w270 w272]
          tunnel: [w269 w273] -> w251
          tunnel: [w268 w272] -> w249
          frame False {
            n121 = Create Folder(path (use dialog)=w271, error in=w270) -> (created path=w269:path, error out=w268:errorcluster)  [unwired: 1 in, 1 out]
          }
          frame True {
          }
        }
        n122 = case shown="True" w259 {
          tunnel: w258 -> [w277 w279]
          tunnel: w257 -> [w276 w278]
          tunnel: [w275 w279] -> w256
          tunnel: [w274 w278] -> w248
          frame False {
            n123 = Create Folder(path (use dialog)=w277, error in=w276) -> (created path=w275:path, error out=w274:errorcluster)  [unwired: 1 in, 1 out]
          }
          frame True {
          }
        }
        n124 = Merge Errors(w249, w248) -> (w247:errorcluster)
        n125 = Bundle By Name(cluster=w262, "local working folder"=w251, "web working folder"=w256) -> (w261:T6)
        n126 = call <vilib>:"Add State(s) to Queue__JKI_lib_State_Machine.vi"("State(s) in (\"\")"=w267) -> ("States Out"=w266:string)  [unwired: 14 in]
      }
      frame "UI: Cursor Set" {
        # "Argument"
        # "Set and Unset Cursor Busy.\n(Usage: \"UI: Cursor Set >> Busy|Idle\")"
        n127 = case shown="\"Idle\", Default" w280 {
          tunnel: w282 -> [w287 w289]
          tunnel: [w286 w288] -> w281
          frame "Idle", Default {
            n128 = call <vilib>:"Unset Busy.vi"("error in (no error)"=w287) -> ("error out"=w286:errorcluster)  [unwired: 10 in]
          }
          frame "Busy" {
            n129 = call <vilib>:"Set Busy.vi"("error in (no error)"=w289) -> ("error out"=w288:errorcluster)  [unwired: 9 in, 1 out]
          }
        }
        n130 = call <vilib>:"Add State(s) to Queue__JKI_lib_State_Machine.vi"("State(s) in (\"\")"=w285) -> ("States Out"=w284:string)  [unwired: 14 in]
      }
      frame "UI: Front Panel State" {
        # "Argument"
        # "Set Front Panel Open or Closed\n(Usage: \"UI: Front Panel State >> Open|Close\")"
        n131 = Unbundle By Name(w292) -> ("Core.Current VI Reference"=w291:refnum<vi>)
        n132 = case shown="\"Open\", \"Standard\", Default" w290 {
          tunnel: w294 -> [w302 w317 w328 w341 w354]
          tunnel: [w304 w318 w330 w343 w356] -> w293
          tunnel: w291 -> [w303 w315 w329 w342 w355]
          frame "Open", "Standard", Default {
            w297 = T1."Standard" ("State")
            n133 = property class="VI"(reference=w303, error in=w302) -> (reference out=w300:refnum<vi>, error out=w301:errorcluster, "FP.State"=w299:T1)
            n134 = Not Equal?(x=w299, y=w297) -> (x != y?=w298:bool)
            n135 = case shown="False" w298 {
              tunnel: [w308 w310] -> w304
              tunnel: w301 -> [w307 w310]
              tunnel: w300 -> [w306 _]
              tunnel: w297 -> [w305 _]
              frame True {
                n136 = invoke class="VI" method="FP.Open"(reference=w306, error in=w307, "Activate"=TRUE, "State"=w305) -> (error out=w308:errorcluster)  [unwired: 1 in, 4 out]
              }
              frame False {
              }
            }
          }
          frame "Close", "Closed" {
            n137 = property class="VI"(reference=w315, error in=w317) -> (reference out=w314:refnum<vi>, error out=w316:errorcluster, "FP.State"=w312:T1)
            n138 = Not Equal?(x=w312, y=T1."Closed" ("Front Panel Window:State")) -> (x != y?=w311:bool)
            n139 = case shown="True" w311 {
              tunnel: [w319 w322] -> w318
              tunnel: w316 -> [w319 w321]
              tunnel: w314 -> [_ w320]
              frame False {
              }
              frame True {
                n140 = invoke class="VI" method="FP.Close"(reference=w320, error in=w321) -> (error out=w322:errorcluster)  [unwired: 1 in, 2 out]
              }
            }
          }
          frame "Hidden", "Hide" {
            w323 = T1."Hidden" ("State")
            n141 = property class="VI"(reference=w329, error in=w328) -> (reference out=w326:refnum<vi>, error out=w327:errorcluster, "FP.State"=w325:T1)
            n142 = Not Equal?(x=w325, y=w323) -> (x != y?=w324:bool)
            n143 = case shown="True" w324 {
              tunnel: [w334 w335] -> w330
              tunnel: w327 -> [w333 w335]
              tunnel: w326 -> [w332 _]
              tunnel: w323 -> [w331 _]
              frame True {
                n144 = invoke class="VI" method="FP.Open"(reference=w332, error in=w333, "State"=w331) -> (error out=w334:errorcluster)  [unwired: 2 in, 4 out]
              }
              frame False {
              }
            }
          }
          frame "Minimize", "Minimized" {
            w336 = T1."Minimized" ("State")
            n145 = property class="VI"(reference=w342, error in=w341) -> (reference out=w339:refnum<vi>, error out=w340:errorcluster, "FP.State"=w338:T1)
            n146 = Not Equal?(x=w338, y=w336) -> (x != y?=w337:bool)
            n147 = case shown="True" w337 {
              tunnel: [w347 w348] -> w343
              tunnel: w340 -> [w346 w348]
              tunnel: w339 -> [w345 _]
              tunnel: w336 -> [w344 _]
              frame True {
                n148 = invoke class="VI" method="FP.Open"(reference=w345, error in=w346, "State"=w344) -> (error out=w347:errorcluster)  [unwired: 2 in, 4 out]
              }
              frame False {
              }
            }
          }
          frame "Maximize", "Maximized" {
            w349 = T1."Maximized" ("State")
            n149 = property class="VI"(reference=w355, error in=w354) -> (reference out=w352:refnum<vi>, error out=w353:errorcluster, "FP.State"=w351:T1)
            n150 = Not Equal?(x=w351, y=w349) -> (x != y?=w350:bool)
            n151 = case shown="True" w350 {
              tunnel: [w360 w361] -> w356
              tunnel: w353 -> [w359 w361]
              tunnel: w352 -> [w358 _]
              tunnel: w349 -> [w357 _]
              frame True {
                n152 = invoke class="VI" method="FP.Open"(reference=w358, error in=w359, "State"=w357) -> (error out=w360:errorcluster)  [unwired: 2 in, 4 out]
              }
              frame False {
              }
            }
          }
        }
        n153 = call <vilib>:"Add State(s) to Queue__JKI_lib_State_Machine.vi"("State(s) in (\"\")"=w296) -> ("States Out"=w295:string)  [unwired: 14 in]
      }
      frame "---------- Macro ----------" {
        # "Do not put any code in this frame.\n(It is a separator no-op. You can make a copy of this frame to create a new Macro frame)"
        n154 = call <vilib>:"Add State(s) to Queue__JKI_lib_State_Machine.vi"("State(s) in (\"\")"=w365) -> ("States Out"=w364:string)  [unwired: 14 in]
      }
      frame "Macro: Display Current" {
        n155 = call <vilib>:"Add State(s) to Queue__JKI_lib_State_Machine.vi"("State(s) in Front (\"\")"="UI: Validate\nActions: Clean local Folder\nActions: Expand cbz\nActions: Display Local Cover", "State(s) in (\"\")"=w370) -> ("States Out"=w369:string)  [unwired: 13 in]
      }
      frame "Macro: Display Web" {
        n156 = call <vilib>:"Add State(s) to Queue__JKI_lib_State_Machine.vi"("State(s) in Front (\"\")"="UI: Validate\nActions: Clean Web Folder\nActions: Download Cover\nActions: Display Web Cover", "State(s) in (\"\")"=w375) -> ("States Out"=w374:string)  [unwired: 13 in]
      }
      frame "Macro: Update UI" {
        n157 = call <vilib>:"Add State(s) to Queue__JKI_lib_State_Machine.vi"("State(s) in Front (\"\")"="UI: Cursor Set >> Busy\nUI: Populate Current\nActions: Load json\nUI: Populate From json\nActions: Check Sync\nActions: Check Size\nUI: Validate\nActions: Find Missing Current\nUI: Cursor Set >> Idle\nUI: Reset Selections", "State(s) in (\"\")"=w380) -> ("States Out"=w379:string)  [unwired: 13 in]
      }
      frame "Macro: Initialize" {
        w381 = "Data: Initialize\nInitialize Core Data\nUI: Initialize\nUI: Front Panel State >> Open"  # Data: Initialize Initialize Core Data UI: Initialize UI: Front Panel State >> Open
        # "Initialization Macro\n(This is called once, when the VI starts)"
        n158 = call <vilib>:"Add State(s) to Queue__JKI_lib_State_Machine.vi"("State(s) in Front (\"\")"=w381, "State(s) in (\"\")"=w385) -> ("States Out"=w384:string)  [unwired: 13 in]
      }
      frame "Macro: Exit" {
        # "Exit Macro\n(This is called once, when the VI exits)"
        n159 = Unbundle By Name(w392) -> ("Core.Close Panel on Exit?"=w391:bool)
        n160 = Select(t="UI: Front Panel State >> Close", s=w391, f="") -> (s? t:f=w388:string)
        n161 = call <vilib>:"Add State(s) to Queue__JKI_lib_State_Machine.vi"("State(s) in (\"\")"=w388, "State(s) at Back (\"\")"="Data: Cleanup\nExit") -> ("States Out"=w386:string)  [unwired: 13 in]
        n162 = call <vilib>:"Add State(s) to Queue__JKI_lib_State_Machine.vi"("State(s) in Front (\"\")"=w386, "State(s) in (\"\")"=w395) -> ("States Out"=w394:string)  [unwired: 13 in]
      }
      frame "---------- Actions ----------" {
        # "Template Separator\n(You can make a copy of, or modify, this frame)"
        n163 = call <vilib>:"Add State(s) to Queue__JKI_lib_State_Machine.vi"("State(s) in (\"\")"=w399) -> ("States Out"=w398:string)  [unwired: 14 in]
      }
      frame "Actions: Open Folder" {
        # "Template Separator\n(You can make a copy of, or modify, this frame)"
        n164 = Unbundle By Name(w403) -> ("current folder"=w402:path)
        n165 = call <vilib>:"Show in File System.vi"("error in (no error)"=w401, "file or directory path"=w402) -> ("error out"=w400:errorcluster)  [unwired: 9 in]
        n166 = call <vilib>:"Add State(s) to Queue__JKI_lib_State_Machine.vi"("State(s) in (\"\")"=w405) -> ("States Out"=w404:string)  [unwired: 14 in]
      }
      frame "Actions: Find Missing Current" {
        n167 = property on="Current" class="LstBox (strict)"() -> ("Item Names"=w422:string[])  [unwired: 2 in, 2 out]
        n168 = property on="From json" class="LstBox (strict)"() -> ("Item Names"=w421:string[])  [unwired: 2 in, 2 out]
        n169 = for {
          tunnel: w422 -> [w474] mode=indexing
          tunnel: [w470] -> w418 mode=indexing
          n170 = call-poly <userlib>:"Strip Path Extension__ogtk.vi"("path"=w474) -> ("root"=w473:string)  [unwired: 1 out]
          n171 = Match Pattern(string=w473, regular expression="#") -> (after substring=w471:string)  [unwired: 1 in, 3 out]
          n172 = Fract/Exp String To Number(string=w471) -> (number=w470:dbl)  [unwired: 3 in, 1 out]
        }
        n173 = for {
          tunnel: w421 -> [w469] mode=indexing
          tunnel: [w465] -> w416 mode=indexing
          n174 = call-poly <userlib>:"Strip Path Extension__ogtk.vi"("path"=w469) -> ("root"=w468:string)  [unwired: 1 out]
          n175 = Match Pattern(string=w468, regular expression="#") -> (after substring=w466:string)  [unwired: 1 in, 3 out]
          n176 = Fract/Exp String To Number(string=w466) -> (number=w465:dbl)  [unwired: 3 in, 1 out]
        }
        n177 = call-poly <userlib>:"Remove Duplicates from 1D Array__ogtk.vi"("Input Array"=w416) -> ("indices of removed elements"=w415:i32[])  [unwired: 1 out]
        n178 = for {
          tunnel: w416 -> [w459] mode=indexing
          tunnel: w418 -> [w461]
          tunnel: [w458] -> w407 mode=indexing if=w457
          n179 = Search 1D Array(1D array=w461, element=w459) -> (index of element=w460:i32)  [unwired: 1 in]
          n180 = case shown="-1" w460 {
            tunnel: w459 -> [_ w463]
            tunnel: [_ w462] -> w458
            tunnel: [_ TRUE] -> w457
            frame Default {
            }
            frame -1 {
              n181 = call "DblToGString.vi"("Numeric"=w463) -> ("String"=w462:string)
            }
          }
        }
        n182 = for {
          tunnel: w418 -> [w451] mode=indexing
          tunnel: w416 -> [w453]
          tunnel: [w450] -> w411 mode=indexing if=w449
          n183 = Search 1D Array(1D array=w453, element=w451) -> (index of element=w452:i32)  [unwired: 1 in]
          n184 = case shown="-1" w452 {
            tunnel: w451 -> [_ w455]
            tunnel: [_ w454] -> w450
            tunnel: [_ TRUE] -> w449
            frame Default {
            }
            frame -1 {
              n185 = call "DblToGString.vi"("Numeric"=w455) -> ("String"=w454:string)
            }
          }
        }
        n186 = for {
          tunnel: w416 -> [w448]
          tunnel: w415 -> [w447] mode=indexing
          tunnel: [w446] -> w409 mode=indexing
          n187 = Index Array(array=w448, index=w447) -> (element=w446:dbl)
        }
        n188 = Empty Array?(array=w409) -> (empty?=w413:bool)
        n189 = Sort 1D Array(array=w409) -> (sorted array=w408:dbl[])
        n190 = Empty Array?(array=w411) -> (empty?=w412:bool)
        n191 = Empty Array?(array=w407) -> (empty?=w414:bool)
        n192 = case shown="False" w413 {
          tunnel: [w436 _] -> w417
          tunnel: w408 -> [w435 _]
          frame False {
            n193 = call "DblToGStringArray.vi"("Array"=w435) -> ("Array 2"=w434:string[])
            n194 = call <userlib>:"1D Array to String__ogtk.vi"("delimiter (Tab)"=", ", "Array of Strings"=w434) -> ("delimited string"=w438:string)  [unwired: 9 in]
            n195 = Format Into String(format string="\\nDuplicates: %s" ("delimiter (Tab)"), w438) -> (resulting string=w436:string)  [unwired: 2 in, 1 out]
          }
          frame True {
          }
        }
        n196 = Sort 1D Array(array=w407) -> (sorted array=w406:string[])
        n197 = Sort 1D Array(array=w411) -> (sorted array=w410:string[])
        n198 = case shown="False" w412 {
          tunnel: [w430 w433] -> w419
          tunnel: w417 -> [w428 w433]
          tunnel: w410 -> [w427 _]
          frame False {
            n199 = call <userlib>:"1D Array to String__ogtk.vi"("delimiter (Tab)"=", ", "Array of Strings"=w427) -> ("delimited string"=w432:string)  [unwired: 9 in]
            n200 = Format Into String(format string="Missing: %s%s" ("delimiter (Tab)"), w432, w428) -> (resulting string=w430:string)  [unwired: 2 in, 1 out]
          }
          frame True {
          }
        }
        "missing json" <- w419
        n201 = case shown="False" w414 {
          tunnel: [w444 "Matching"] -> w420
          tunnel: w406 -> [w443 _]
          frame False {
            n202 = call <userlib>:"1D Array to String__ogtk.vi"("delimiter (Tab)"=", ", "Array of Strings"=w443) -> ("delimited string"=w441:string)  [unwired: 9 in]
            n203 = Format Into String(format string="Missing: %s" ("delimiter (Tab)"), w441) -> (resulting string=w444:string)  [unwired: 2 in, 1 out]
          }
          frame True {
          }
        }
        "missing current" <- w420
        n204 = call <vilib>:"Add State(s) to Queue__JKI_lib_State_Machine.vi"("State(s) in (\"\")"=w426) -> ("States Out"=w425:string)  [unwired: 14 in]
      }
      frame "Actions: Create New Folder" {
        # "Template Separator\n(You can make a copy of, or modify, this frame)"
        n205 = call-poly <userlib>:"Strip Path Extension__ogtk.vi"("path"="json file path") -> ("extension"=w483:string)  [unwired: 1 out]
        n206 = call <vilib>:"Check if File or Folder Exists.vi"("error in (no error)"=w478, "path"="json file path") -> ("error out"=w479:errorcluster, "file or folder exists?"=w476:bool, "dup path"=w480:path)  [unwired: 7 in]
        n207 = Equal?(x="json", y=w483) -> (x = y?=w477:bool)
        n208 = And(x=w477, y=w476) -> (x .and. y?=w475:bool)
        n209 = case shown="True" w475 {
          tunnel: [w488 w491] -> w484
          tunnel: w480 -> [_ w490]
          tunnel: w479 -> [w488 w489]
          frame False {
          }
          frame True {
            n210 = call "CreateFolderFromJSON.vi"("error in"=w489, "json file path"=w490) -> ("error out"=w491:errorcluster)  [unwired: 9 in]
          }
        }
        n211 = call <vilib>:"Add State(s) to Queue__JKI_lib_State_Machine.vi"("State(s) in (\"\")"=w487) -> ("States Out"=w486:string)  [unwired: 14 in]
      }
      frame "Actions: Delete from json" {
        n212 = Unbundle By Name(w513) -> ("comic jsons"=w516:T5[], "current folder"=w511:path)
        n213 = local read "From json"() -> (w515:i32)
        n214 = call <vilib>:"Recursive File List.vi"("pattern"="comics.*.json", "error in (no error)"=w509, "Folder Path"=w511) -> ("error out"=w507:errorcluster, "All Files in Dir"=w508:path[])  [unwired: 4 in, 3 out]
        n215 = Index Array(array=w508) -> (element=w503:path)  [unwired: 1 in]
        n216 = Delete From Array(array=w516, length=1, index=w515) -> (array with subset deleted=w506:T5[])  [unwired: 1 out]
        n217 = Read from Text File(file (use dialog)=w503, error in=w507) -> (text=w492:string, error out=w495:errorcluster)  [unwired: 2 in, 2 out]
        n218 = call "parse.comics_reply.vi"("error in"=w495, "string in"=w492) -> ("error out"=w494:errorcluster, "data"=w493:T8)  [unwired: 8 in]
        n219 = Bundle By Name(cluster=w513, "comic jsons"=w506) -> (w512:T6)
        n220 = Bundle By Name(cluster=w493, "data.results"=w506) -> (w505:T8)
        n221 = call <vilib>:"Flatten To JSON String.vi"("error in (no error)"=w494, "Variant"=w505) -> ("error out"=w504:errorcluster, "JSON String"=w499:string)  [unwired: 8 in]
        n222 = Open/Create/Replace File(file path (use dialog)=w503, error in=w504, operation (0:open)=T3."replace") -> (refnum out=w500:refnum<file>, error out=w501:errorcluster)  [unwired: 3 in, 1 out]
        n223 = Write to Text File(file (use dialog)=w500, text=w499, error in=w501) -> (refnum out=w497:refnum<file>, error out=w498:errorcluster)  [unwired: 1 in, 1 out]
        n224 = Close File(refnum=w497, error in=w498) -> (error out=w496:errorcluster)  [unwired: 1 out]
        n225 = call <vilib>:"Add State(s) to Queue__JKI_lib_State_Machine.vi"("State(s) in (\"\")"=w518) -> ("States Out"=w517:string)  [unwired: 14 in]
      }
      frame "Actions: Rename json title" {
        n226 = call "Enter New Filename"("error in (no error)"=w522) -> ("New filename"=w519:string, "OK"=w520:bool, "error out"=w521:errorcluster)  [unwired: 16 in]
        n227 = case shown="True" w520 {
          tunnel: w525 -> [w528 w530]
          tunnel: [w528 w554] -> w524
          tunnel: [w529 w540] -> w523
          tunnel: w521 -> [w529 w535]
          tunnel: w519 -> [_ w531]
          frame False {
          }
          frame True {
            n228 = Unbundle By Name(w530) -> ("comic jsons"=w534:T5[], "current folder"=w553:path)
            n229 = local read "From json"() -> (w532:i32)
            n230 = call <vilib>:"Recursive File List.vi"("pattern"="comics.*.json", "error in (no error)"=w535, "Folder Path"=w553) -> ("error out"=w550:errorcluster, "All Files in Dir"=w551:path[])  [unwired: 4 in, 3 out]
            n231 = call "rename.single.title.vi"("index"=w532, "title"=w531, "comic jsons"=w534) -> ("comic jsons 2"=w533:T5[])  [unwired: 8 in]
            n232 = Index Array(array=w551) -> (element=w547:path)  [unwired: 1 in]
            n233 = Read from Text File(file (use dialog)=w547, error in=w550) -> (text=w536:string, error out=w539:errorcluster)  [unwired: 2 in, 2 out]
            n234 = Bundle By Name(cluster=w530, "comic jsons"=w533) -> (w554:T6)
            n235 = call "parse.comics_reply.vi"("error in"=w539, "string in"=w536) -> ("error out"=w538:errorcluster, "data"=w537:T8)  [unwired: 8 in]
            n236 = Bundle By Name(cluster=w537, "data.results"=w533) -> (w549:T8)
            n237 = call <vilib>:"Flatten To JSON String.vi"("error in (no error)"=w538, "Variant"=w549) -> ("error out"=w548:errorcluster, "JSON String"=w543:string)  [unwired: 8 in]
            n238 = Open/Create/Replace File(file path (use dialog)=w547, error in=w548, operation (0:open)=T3."replace") -> (refnum out=w544:refnum<file>, error out=w545:errorcluster)  [unwired: 3 in, 1 out]
            n239 = Write to Text File(file (use dialog)=w544, text=w543, error in=w545) -> (refnum out=w541:refnum<file>, error out=w542:errorcluster)  [unwired: 1 in, 1 out]
            n240 = Close File(refnum=w541, error in=w542) -> (error out=w540:errorcluster)  [unwired: 1 out]
          }
        }
        n241 = call <vilib>:"Add State(s) to Queue__JKI_lib_State_Machine.vi"("State(s) in (\"\")"=w527) -> ("States Out"=w526:string)  [unwired: 14 in]
      }
      frame "Actions: Download Cover" {
        n242 = Unbundle By Name(w558) -> ("json present"=w561:bool, "web working folder"=w563:path, "comic jsons"=w565:T5[])
        n243 = local read "From json"() -> (w564:i32)
        n244 = case shown="True" w561 {
          tunnel: w565 -> [_ w588]
          tunnel: w564 -> [_ w587]
          tunnel: w563 -> [_ w581]
          tunnel: w562 -> [w573 w578]
          tunnel: [w573 w577] -> w560
          tunnel: [_ TRUE] -> w555
          frame False {
          }
          frame True {
            n245 = Index Array(array=w588, index=w587) -> (element=w586:T5)
            n246 = Unbundle By Name(w586) -> ("images"=w585:cluster{"path":string, "extension":string}[])
            n247 = Build Path(base path=w581, name or relative path=path "temp.jpg") -> (appended path=w579:path)
            n248 = Index Array(array=w585) -> (element=w584:cluster{"path":string, "extension":string})  [unwired: 1 in]
            n249 = Unbundle By Name(w584) -> ("path"=w583:string, "extension"=w576:string)
            n250 = Concatenate Strings(w583, "." ("string"), w576) -> (w582:string)
            n251 = call <vilib>:"GET.vi"("output file"=w579, "url"=w582, "error in (no error)"=w578) -> ("error out"=w577:errorcluster)  [unwired: 9 in, 3 out]
          }
        }
        n252 = case shown="Error 59" w560 {
          selector: w560 -> [w569 w570 w572]
          tunnel: [w569 w570 w571] -> w559
          tunnel: [w568 _ _] -> w556
          tunnel: w555 -> [w568 _ _]
          frame No Error {
          }
          frame Default {
          }
          frame Error {
            n253 = call <vilib>:"Clear Errors.vi"("error in (no error)"=w572) -> ("error out"=w571:errorcluster)  [unwired: 5 in, 1 out]
          }
        }
        n254 = Bundle By Name(cluster=w558, "display web"=w556) -> (w557:T6)
        n255 = call <vilib>:"Add State(s) to Queue__JKI_lib_State_Machine.vi"("State(s) in (\"\")"=w567) -> ("States Out"=w566:string)  [unwired: 14 in]
      }
      frame "Actions: Display Local Cover" {
        n256 = Unbundle By Name(w610) -> ("local working folder"=w609:path)
        n257 = List Folder(path=w609, error in=w608) -> (path out=w606:path, filenames=w607:string[], error out=w605:errorcluster)  [unwired: 2 in, 1 out]
        n258 = Index Array(array=w607) -> (element=w590:string)  [unwired: 1 in]
        n259 = Build Path(base path=w606, name or relative path=w590) -> (appended path=w591:path)
        n260 = call-poly <userlib>:"Strip Path Extension__ogtk.vi"("path"=w590) -> ("extension"=w589:string)  [unwired: 1 out]
        n261 = case shown="\"jpeg\", \"jpg\"" w589 {
          tunnel: w605 -> [w613 w618 w623]
          tunnel: [_ w617 w622] -> w598
          tunnel: [_ w616 w621] -> w596
          tunnel: [w613 w615 w620] -> w594
          tunnel: w591 -> [_ w614 w619]
          frame Default {
          }
          frame "jpeg", "jpg" {
            n262 = call <vilib>:"Read JPEG File.vi"("error in (no error)"=w618, "path to JPEG file"=w614) -> ("error out"=w615:errorcluster, "image data"=w616:T9)  [unwired: 7 in, 1 out]
            n263 = call <vilib>:"Draw Flattened Pixmap.vi"("image data"=w616) -> ("new picture"=w617:picture)  [unwired: 8 in]
          }
          frame "png" {
            n264 = call <vilib>:"Read PNG File.vi"("error in (no error)"=w623, "path to PNG file"=w619) -> ("error out"=w620:errorcluster, "image data"=w621:T9)  [unwired: 7 in, 1 out]
            n265 = call <vilib>:"Draw Flattened Pixmap.vi"("image data"=w621) -> ("new picture"=w622:picture)  [unwired: 8 in]
          }
        }
        "Local Cover" <- w598
        n266 = property on="Local Cover" class="Pict"(error in=w594) -> (error out=w593:errorcluster, "Draw Area Size"=w597:T10)  [unwired: 1 in, 1 out]
        n267 = Unbundle By Name(w596) -> ("Rectangle.right"=w602:i16, "Rectangle.bottom"=w601:i16)
        n268 = Unbundle By Name(w597) -> ("Width"=w604:u32, "Height"=w603:u32)
        n269 = Divide(x=w604, y=w602) -> (x/y=w600:dbl)
        n270 = Divide(x=w603, y=w601) -> (x/y=w599:dbl)
        n271 = Max & Min(x=w600, y=w599) -> (min(x,y)=w595:dbl)  [unwired: 1 out]
        n272 = property on="Local Cover" class="Pict"(error in=w593, "ZoomFactor"=w595) -> (error out=w592:errorcluster)  [unwired: 1 in, 1 out]
        n273 = call <vilib>:"Add State(s) to Queue__JKI_lib_State_Machine.vi"("State(s) in (\"\")"=w612) -> ("States Out"=w611:string)  [unwired: 14 in]
      }
      frame "Actions: Display Web Cover" {
        n274 = Unbundle By Name(w643) -> ("web working folder"=w628:path, "json present"=w626:bool, "display web"=w625:bool)
        "Available?" <- w625
        n275 = And(x=w626, y=w625) -> (x .and. y?=w627:bool)
        n276 = case shown="True" w627 {
          tunnel: [_ w652] -> w635
          tunnel: [w646 w651] -> w633
          tunnel: [_ w650] -> w630
          tunnel: w629 -> [w646 w649]
          tunnel: w628 -> [_ w648]
          tunnel: path "temp.jpg" ("name or relative path") -> [_ w647]
          frame False {
          }
          frame True {
            n277 = Build Path(base path=w648, name or relative path=w647) -> (appended path=w653:path)
            n278 = call <vilib>:"Read JPEG File.vi"("error in (no error)"=w649, "path to JPEG file"=w653) -> ("error out"=w651:errorcluster, "image data"=w652:T9)  [unwired: 7 in, 1 out]
            n279 = call <vilib>:"Draw Flattened Pixmap.vi"("image data"=w652) -> ("new picture"=w650:picture)  [unwired: 8 in]
          }
        }
        "web cover" <- w630
        n280 = property on="web cover" class="Pict"(error in=w633) -> (error out=w632:errorcluster, "Draw Area Size"=w636:T10)  [unwired: 1 in, 1 out]
        n281 = Unbundle By Name(w635) -> ("Rectangle.right"=w640:i16, "Rectangle.bottom"=w639:i16)
        n282 = Unbundle By Name(w636) -> ("Width"=w642:u32, "Height"=w641:u32)
        n283 = Divide(x=w642, y=w640) -> (x/y=w638:dbl)
        n284 = Divide(x=w641, y=w639) -> (x/y=w637:dbl)
        n285 = Max & Min(x=w638, y=w637) -> (min(x,y)=w634:dbl)  [unwired: 1 out]
        n286 = property on="web cover" class="Pict"(error in=w632, "ZoomFactor"=w634) -> (error out=w631:errorcluster)  [unwired: 1 in, 1 out]
        n287 = call <vilib>:"Add State(s) to Queue__JKI_lib_State_Machine.vi"("State(s) in (\"\")"=w645) -> ("States Out"=w644:string)  [unwired: 14 in]
      }
      frame "Actions: Expand cbz" {
        n288 = Unbundle By Name(w662) -> ("current folder"=w656:path, "local working folder"=w661:path)
        n289 = property on="Current" class="LstBox (strict)"(error in=w658) -> (error out=w654:errorcluster, "Item Names"=w659:string[], "Value"=w660:i32)  [unwired: 1 in, 1 out]
        n290 = Index Array(array=w659, index=w660) -> (element=w657:string)
        n291 = Build Path(base path=w656, name or relative path=w657) -> (appended path=w655:path)
        n292 = call "PathToQuotedString.vi"("Path"=w661) -> ("String"=w666:string)  [unwired: 10 in]
        n293 = call "PathToQuotedString.vi"("Path"=w655) -> ("String"=w665:string)  [unwired: 10 in]
        n294 = Format Into String(format string="%s e %s -o%s -r", error in=w654, "\"C:\\Program Files\\7-Zip\\7z.exe\"" ("input 1"), w665, w666) -> (resulting string=w668:string, error out=w669:errorcluster)  [unwired: 1 in]
        n295 = call <vilib>:"System Exec.vi"("run minimized? (F)"=TRUE, "error in (no error)"=w669, "command line"=w668) -> ("error out"=w663:errorcluster)  [unwired: 5 in, 3 out]
        n296 = call <vilib>:"Add State(s) to Queue__JKI_lib_State_Machine.vi"("State(s) in (\"\")"=w672) -> ("States Out"=w671:string)  [unwired: 14 in]
      }
      frame "Actions: Clean local folder" {
        n297 = Unbundle By Name(w674) -> ("local working folder"=w673:path)
        n298 = call "ClearWorkingDirectory.vi"("error in"=w675, "Working Path"=w673) -> ("error out"=w676:errorcluster)  [unwired: 8 in, 1 out]
        n299 = call <vilib>:"Add State(s) to Queue__JKI_lib_State_Machine.vi"("State(s) in (\"\")"=w678) -> ("States Out"=w677:string)  [unwired: 14 in]
      }
      frame "Actions: Clean Web Folder" {
        n300 = Unbundle By Name(w680) -> ("web working folder"=w679:path)
        n301 = call "ClearWorkingDirectory.vi"("error in"=w681, "Working Path"=w679) -> ("error out"=w682:errorcluster)  [unwired: 8 in, 1 out]
        n302 = call <vilib>:"Add State(s) to Queue__JKI_lib_State_Machine.vi"("State(s) in (\"\")"=w684) -> ("States Out"=w683:string)  [unwired: 14 in]
      }
      frame "Actions: Load json" {
        # "Template Separator\n(You can make a copy of, or modify, this frame)"
        n303 = Unbundle By Name(w693) -> ("current folder"=w700:path)
        n304 = List Folder(path=w700, pattern="comics.*.json", error in=w695) -> (path out=w696:path, filenames=w698:string[], error out=w690:errorcluster)  [unwired: 1 in, 1 out]
        n305 = Index Array(array=w698) -> (element=w697:string)  [unwired: 1 in]
        n306 = Build Path(base path=w696, name or relative path=w697) -> (appended path=w688:path)
        n307 = call <vilib>:"Check if File or Folder Exists.vi"("error in (no error)"=w690, "path"=w688) -> ("error out"=w689:errorcluster, "file or folder exists?"=w686:bool, "dup path"=w687:path)  [unwired: 7 in]
        n308 = case shown="True" w686 {
          selector: w686 -> [w703 w705]
          tunnel: [w704 w709] -> w694
          tunnel: [_ w708] -> w691
          tunnel: w689 -> [w704 w707]
          tunnel: w687 -> [_ w706]
          tunnel: [w703 w705] -> w685
          frame False {
          }
          frame True {
            n309 = Read from Text File(file (use dialog)=w706, error in=w707) -> (text=w712:string, error out=w711:errorcluster)  [unwired: 2 in, 2 out]
            n310 = call "parse.comics_reply.vi"("error in"=w711, "string in"=w712) -> ("error out"=w709:errorcluster, "data"=w710:T8)  [unwired: 8 in]
            n311 = Unbundle By Name(w710) -> ("data.results"=w708:T5[])
          }
        }
        n312 = Bundle By Name(cluster=w693, "json present"=w685, "comic jsons"=w691) -> (w692:T6)
        n313 = call <vilib>:"Add State(s) to Queue__JKI_lib_State_Machine.vi"("State(s) in (\"\")"=w702) -> ("States Out"=w701:string)  [unwired: 14 in]
      }
      frame "Actions: Check Size" {
        # "Template Separator\n(You can make a copy of, or modify, this frame)"
        n314 = Unbundle By Name(w715) -> ("json present"=w714:bool)
        n315 = case shown="True" w714 {
          tunnel: w719 -> [w723 w735]
          tunnel: [T4."Disabled and Grayed Out" ("Disabled") w726] -> w718
          tunnel: [w723 w725] -> w717
          tunnel: [_ w724] -> w713
          frame False {
          }
          frame True {
            n316 = property on="Current" class="LstBox (strict)"(error in=w735) -> (error out=w730:errorcluster, "Item Names"=w734:string[])  [unwired: 1 in, 1 out]
            n317 = property on="From json" class="LstBox (strict)"(error in=w735) -> (error out=w729:errorcluster, "Item Names"=w733:string[])  [unwired: 1 in, 1 out]
            n318 = Array Size(array=w734) -> (size(s)=w732:i32)
            n319 = Array Size(array=w733) -> (size(s)=w731:i32)
            n320 = Merge Errors(w730, w729) -> (w725:errorcluster)
            n321 = Equal?(x=w732, y=w731) -> (x = y?=w724:bool)
            n322 = Select(t=T4."Enabled" ("Disabled"), s=w724, f=T4."Disabled and Grayed Out" ("Disabled")) -> (s? t:f=w726:T4)
          }
        }
        "totals match" <- w713
        n323 = property on="Rename All" class="Bool"(error in=w717, "DisabledEnum"=w718) -> (error out=w716:errorcluster)  [unwired: 1 in, 1 out]
        n324 = call <vilib>:"Add State(s) to Queue__JKI_lib_State_Machine.vi"("State(s) in (\"\")"=w721) -> ("States Out"=w720:string)  [unwired: 14 in]
      }
      frame "Actions: Check Sync" {
        n325 = Unbundle By Name(w738) -> ("json present"=w736:bool)
        n326 = case shown="False" w736 {
          tunnel: [_ w751] -> w742
          tunnel: [w745 w750] -> w741
          tunnel: [w745 w749] -> w740
          tunnel: w737 -> [w745 w746]
          frame False {
          }
          frame True {
            n327 = property on="Current" class="LstBox (strict)"(error in=w746) -> (error out=w750:errorcluster, "Item Names"=w747:string[])  [unwired: 1 in, 1 out]
            n328 = property on="From json" class="LstBox (strict)"(error in=w746) -> (error out=w749:errorcluster, "Item Names"=w748:string[])  [unwired: 1 in, 1 out]
            n329 = Equal?(x=w747, y=w748) -> (x = y?=w751:bool)
          }
        }
        "synced" <- w742
        n330 = Merge Errors(w741, w740) -> (w739:errorcluster)
        n331 = call <vilib>:"Add State(s) to Queue__JKI_lib_State_Machine.vi"("State(s) in (\"\")"=w744) -> ("States Out"=w743:string)  [unwired: 14 in]
      }
      frame "Actions: Rename Selected" {
        n332 = Unbundle By Name(w755) -> ("current folder"=w754:path, "json present"=w752:bool)
        n333 = case shown="True" w752 {
          tunnel: w756 -> [w759 w766]
          tunnel: w754 -> [_ w764]
          tunnel: [w759 w761] -> w753
          frame False {
          }
          frame True {
            n334 = local read "From json"() -> (w772:i32)
            n335 = property on="Current" class="LstBox (strict)"(error in=w766) -> (error out=w768:errorcluster, "Item Names"=w771:string[])  [unwired: 1 in, 1 out]
            n336 = property on="From json" class="LstBox (strict)"(error in=w766) -> (error out=w769:errorcluster, "Item Names"=w773:string[])  [unwired: 1 in, 1 out]
            n337 = local read "Current"() -> (w770:i32)
            n338 = Index Array(array=w771, index=w770) -> (element=w765:string)
            n339 = Merge Errors(w768, w769) -> (w767:errorcluster)
            n340 = Index Array(array=w773, index=w772) -> (element=w760:string)
            n341 = Build Path(base path=w764, name or relative path=w765) -> (appended path=w762:path)
            n342 = Build Path(base path=w764, name or relative path=w760) -> (appended path=w763:path)
            n343 = Move(source path=w762, error in=w767, 10:w763) -> (error out=w761:errorcluster)  [unwired: 2 in, 2 out]
          }
        }
        n344 = call <vilib>:"Add State(s) to Queue__JKI_lib_State_Machine.vi"("State(s) in (\"\")"=w758) -> ("States Out"=w757:string)  [unwired: 14 in]
      }
      frame "Actions: Rename All" {
        n345 = Unbundle By Name(w777) -> ("current folder"=w776:path, "json present"=w774:bool)
        n346 = case shown="True" w774 {
          tunnel: w778 -> [w781 w784]
          tunnel: w776 -> [_ w783]
          tunnel: [w781 w782] -> w775
          frame False {
          }
          frame True {
            n347 = property on="Current" class="LstBox (strict)"(error in=w784) -> (error out=w786:errorcluster, "Item Names"=w788:string[])  [unwired: 1 in, 1 out]
            n348 = property on="From json" class="LstBox (strict)"(error in=w784) -> (error out=w787:errorcluster, "Item Names"=w789:string[])  [unwired: 1 in, 1 out]
            n349 = Merge Errors(w786, w787) -> (w785:errorcluster)
            n350 = for {
              tunnel: w789 -> [w790] mode=indexing
              tunnel: w788 -> [w794] mode=indexing
              tunnel: w783 -> [w796]
              shift-right: [w795] -> w782
              shift-left: w785 -> [w797]
              n351 = Build Path(base path=w796, name or relative path=w794) -> (appended path=w793:path)
              n352 = Build Path(base path=w796, name or relative path=w790) -> (appended path=w792:path)
              n353 = Not Equal?(x=w792, y=w793) -> (x != y?=w791:bool)
              n354 = case shown="True" w791 {
                tunnel: w797 -> [w798 w802]
                tunnel: [w798 w801] -> w795
                tunnel: w793 -> [_ w800]
                tunnel: w792 -> [_ w799]
                frame False {
                }
                frame True {
                  n355 = Move(source path=w800, error in=w802, 10:w799) -> (error out=w801:errorcluster)  [unwired: 2 in, 2 out]
                }
              }
            }
          }
        }
        n356 = call <vilib>:"Add State(s) to Queue__JKI_lib_State_Machine.vi"("State(s) in (\"\")"=w780) -> ("States Out"=w779:string)  [unwired: 14 in]
      }
    }
  }
